vi "FPGA_TEST_RampLoop.vi"(6 "edge detected":bool, 9 "direction increment":i32, 10 "total number of ramps":i32, 11 "reset_ramp_x":bool) -> (1 "MaxNoRamp":bool, 2 "DisplacementFinished":bool, 3 "Ramp index":cluster{"ramp index":i32, "NextRamp":i32})   [LabVIEW 2016]
uses:
  <vilib>/Platform/TimedLoop/XDataNode/timing_clust.ctl
  <vilib>/Platform/TimedLoop/XDataNode/nitl_modes.ctl
  <vilib>/Platform/TimedLoop/XDataNode/wakeup.ctl
  <vilib>/rvi/Emulation/niFpgaSctlEmulationGetInTimedLoop.vi
  <vilib>/rvi/Emulation/niFpgaEmulationReportErrorSimple.vi
  <vilib>/rvi/Emulation/niFpgaGetClockAttributes.vi
  <vilib>/rvi/Emulation/niFpgaCriticalErrorInLSC.vi
  <vilib>/platform/TimedLoop/XDataNode/XDataNode.xnode
  <vilib>/Platform/TimedLoop/XDataNode/XDNodeRunTimeDep.lvlib
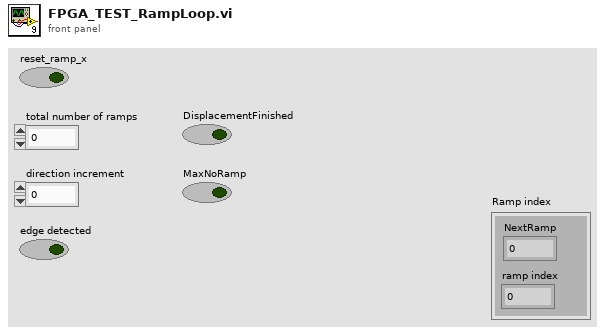
[diagram p1: front panel]
types:
  T1 = typedef "XDNodeRunTimeDep.lvlib/timing_clust.ctl" = cluster{"Expected End [f-1]":u64, "Actual End [f-1]":u64, "Finished Late? [f-1]":bool, "Expected End [i-1]":u64, "Actual End [i-1]":u64, "Finished Late? [i-1]":bool, "Expected Start [i]":u64, "Actual Start [i]":u64, "Expected Start [f]":u64, "Actual Start [f]":u64, "Source Name":string, "Structure Name":string, "Period":i64, "Deadline":i64, "Offset":i64, "Start":i64, "Priority":i32, "Timeout":i32, "Mode":T2, "Wakeup Reason":T3, "Error":errorcluster, "Source Type":string, "Secondary Source Type":string, "Global End Time":u64, "Global Start Time":u64, "Frame Duration":u64, "Iteration Duration":u64, "Assigned CPU":i32, "I/O Scan Engine Mode":u32}
  T2 = typedef "XDNodeRunTimeDep.lvlib/nitl_modes.ctl" = enum32{"No Change", "Process missed periods, maintain original phase", "Discard missed periods, maintain original phase", "Process missed periods, ignore original phase", "Discard missed periods, ignore original phase"}
  T3 = typedef "XDNodeRunTimeDep.lvlib/wakeup.ctl" = enum32{"Normal", "Aborted", "Asynchronous wakeup", "Timing source error", "Timed loop error", "Timeout"}
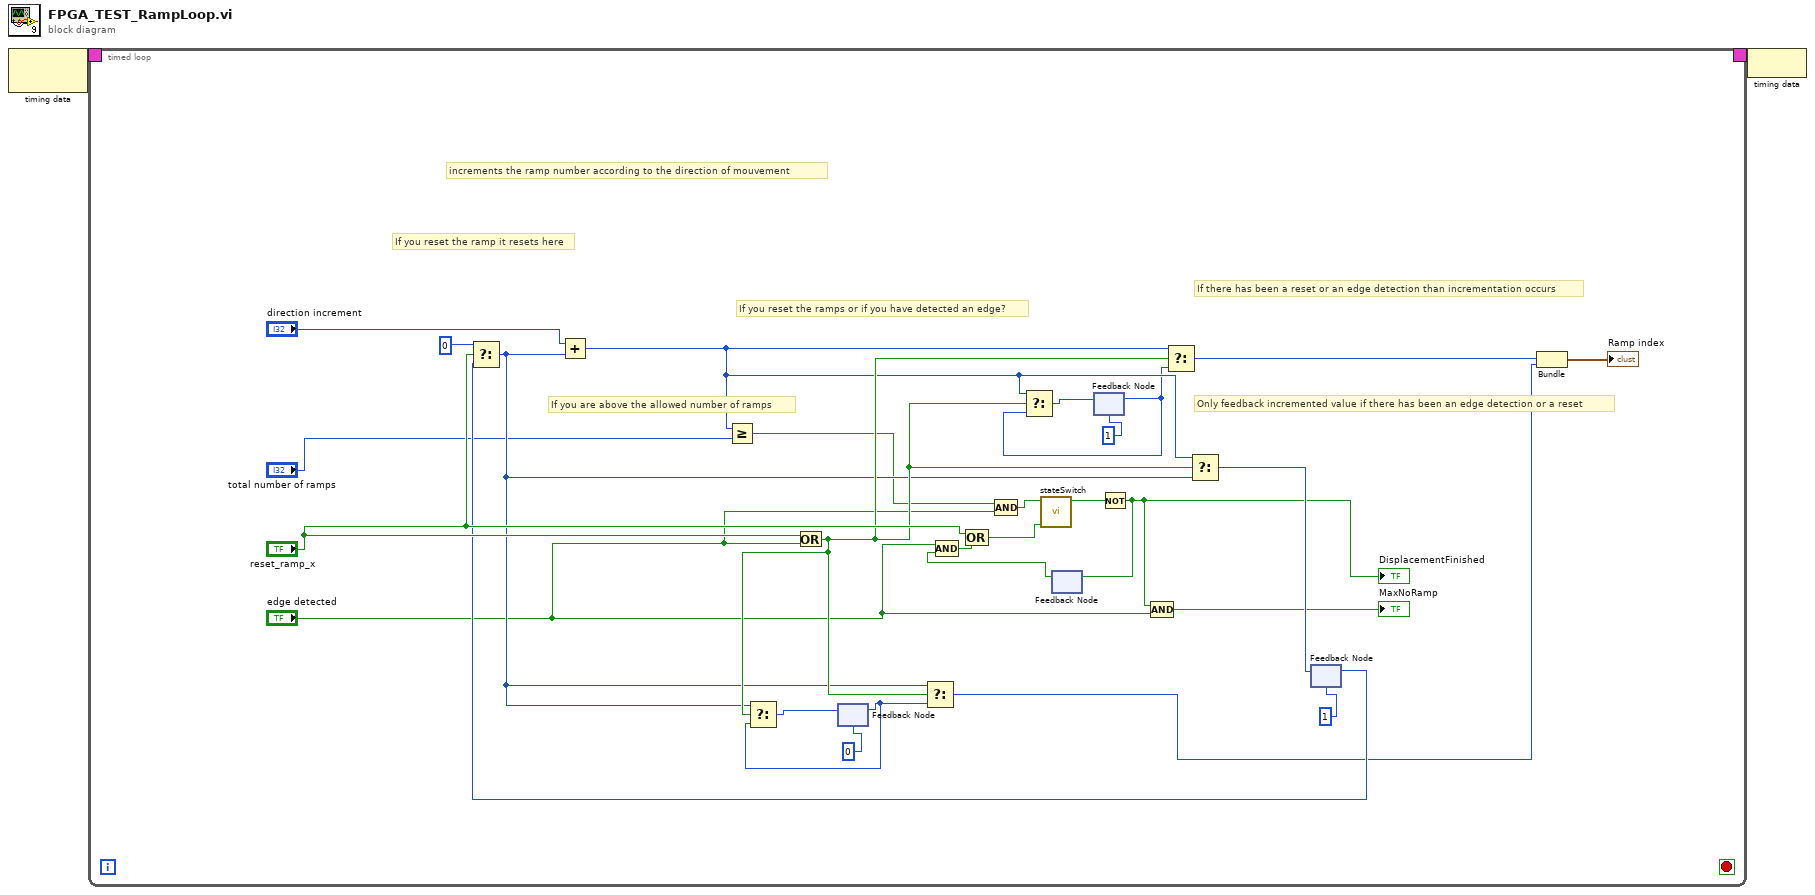
[diagram p0: block diagram]
diagram:
  n1 = node-c288() -> (w2:T1)  [unwired: 1 in]
  n2 = timed-loop {
    timing: w2 -> [_]
    timing-out: [_] -> w1
    stop <- _ stop-if-true
    # "Only feedback incremented value if there has been an edge detection or a reset"
    # "If there has been a reset or an edge detection than incrementation occurs"
    # "If you reset the ramps or if you have detected an edge?"
    # "If you are above the allowed number of ramps"
    # "If you reset the ramp it resets here"
    # "increments the ramp number according to the direction of mouvement"
    n3 = Or(x="reset_ramp_x", y="edge detected") -> (x .or. y?=w26:bool)
    n4 = feedback #1(i16 0) -> (w28:i32)
    n5 = feedback #2() -> (w13:bool)  [unwired: 1 in]
    n6 = Compound Arithmetic op=AND("edge detected", w13) -> (w12:bool)
    n7 = Compound Arithmetic op=OR("reset_ramp_x", w12) -> (w14:bool)
    n8 = feedback #3(i16 1) -> (w19:i32)
    n9 = feedback #4(i16 1) -> (w22:i32)
    n10 = Select(t=i16 0, s="reset_ramp_x", f=w22) -> (s? t:f=w25:i32)
    n11 = Add(x="direction increment", y=w25) -> (x+y=w23:i32)
    n12 = Greater Or Equal?(x=w23, y="total number of ramps") -> (x >= y?=w9:bool)
    n13 = Select(t=w25, s=w26, f=w28) -> (s? t:f=w29:i32)
    n14 = feedback-in #1(w29) -> ()
    n15 = Select(t=w25, s=w26, f=w28) -> (s? t:f=w4:i32)
    n16 = Compound Arithmetic op=AND(w9, "edge detected") -> (w10:bool)
    n17 = Select(t=w23, s=w26, f=w19) -> (s? t:f=w18:i32)
    n18 = call "stateSwitch.vi"("disable"=w14, "enable"=w10) -> ("state"=w11:bool)  [unwired: 9 in]
    n19 = feedback-in #3(w18) -> ()
    n20 = Not(x=w11) -> (.not. x?=w15:bool)
    "DisplacementFinished" <- w15
    n21 = feedback-in #2(w15) -> ()
    n22 = Compound Arithmetic op=AND(w15, "edge detected") -> (→"MaxNoRamp":bool)
    n23 = Select(t=w23, s=w26, f=w19) -> (s? t:f=w5:i32)
    n24 = Select(t=w23, s=w26, f=w25) -> (s? t:f=w24:i32)
    n25 = feedback-in #4(w24) -> ()
    n26 = Bundle(w5, w4) -> (→"Ramp index":cluster{i32, i32})  [unwired: 1 in]
  }
  n27 = node-c288(w1) -> ()
